vi "PathSettings.vi"() -> ()   [LabVIEW 2010]
uses:
  <vilib>/Utility/config.llb/NI_LVConfig.lvlib
  <vilib>/Utility/config.llb/Read Key (String).vi
panel:
  out "Result: XML Footer":string
  out "Result: XML Header":string
  out "Indicator TAG":string
  out "Control TAG":string
  out "Experiment VI":string
  out "Database":string
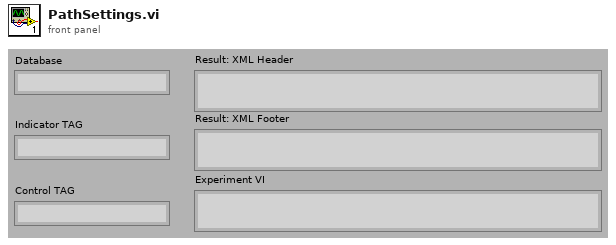
[diagram p1: front panel]
types:
  T1 = typedef "NI_LVConfig.lvlib/Config Data RefNum.ctl" = refnum<k1>
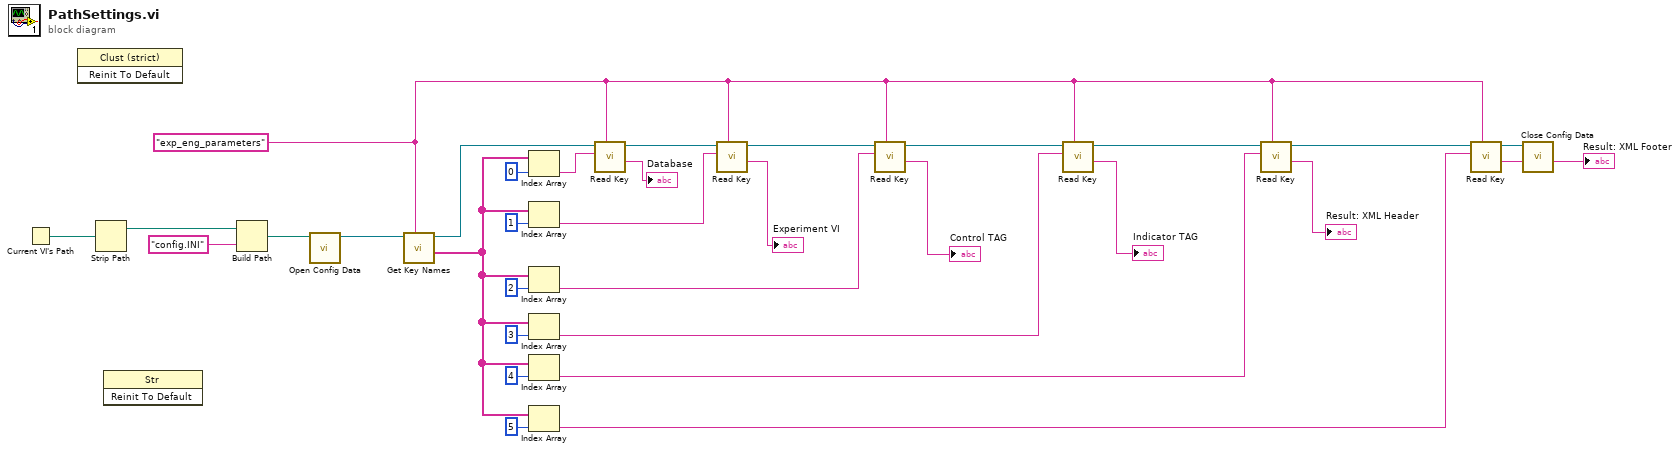
[diagram p0: block diagram]
diagram:
  w9 = "exp_eng_parameters" ("section")
  n1 = Current VI's Path() -> (path=w32:path)
  n2 = invoke on="Invoke Node" class="Clust (strict)" method="Reinit To Default"() -> ()  [unwired: 3 in, 3 out]
  n3 = Strip Path(path=w32) -> (stripped path=w31:path)  [unwired: 1 out]
  n4 = invoke on="Invoke Node" class="Str" method="Reinit To Default"() -> ()  [unwired: 3 in, 3 out]
  n5 = Build Path(base path=w31, name or relative path="config.INI") -> (appended path=w30:path)
  n6 = call <vilib>:"Open Config Data.vi"("configuration file path"=w30) -> ("refnum"=w28:T1)  [unwired: 8 in, 2 out]
  n7 = call <vilib>:"Get Key Names.vi"("section"=w9, "refnum"=w28) -> ("key names"=w11:string[], "refnum out"=w27:T1)  [unwired: 6 in, 2 out]
  n8 = Index Array(array=w11, index=0) -> (element=w25:string)
  n9 = Index Array(array=w11, index=1) -> (element=w23:string)
  n10 = Index Array(array=w11, index=2) -> (element=w19:string)
  n11 = Index Array(array=w11, index=3) -> (element=w16:string)
  n12 = Index Array(array=w11, index=4) -> (element=w14:string)
  n13 = Index Array(array=w11, index=5) -> (element=w10:string)
  n14 = call-poly <vilib>:"Read Key.vi"("section"=w9, "key"=w25, "refnum"=w27) -> ("value"=→"Database":string, "refnum out"=w22:T1)  [unwired: 5 in, 2 out]
  n15 = call-poly <vilib>:"Read Key.vi"("section"=w9, "key"=w23, "refnum"=w22) -> ("value"=→"Experiment VI":string, "refnum out"=w20:T1)  [unwired: 5 in, 2 out]
  n16 = call-poly <vilib>:"Read Key.vi"("section"=w9, "key"=w19, "refnum"=w20) -> ("value"=→"Control TAG":string, "refnum out"=w17:T1)  [unwired: 5 in, 2 out]
  n17 = call-poly <vilib>:"Read Key.vi"("section"=w9, "key"=w16, "refnum"=w17) -> ("value"=→"Indicator TAG":string, "refnum out"=w13:T1)  [unwired: 5 in, 2 out]
  n18 = call-poly <vilib>:"Read Key.vi"("section"=w9, "key"=w14, "refnum"=w13) -> ("value"=→"Result: XML Header":string, "refnum out"=w8:T1)  [unwired: 5 in, 2 out]
  n19 = call-poly <vilib>:"Read Key.vi"("section"=w9, "key"=w10, "refnum"=w8) -> ("value"=→"Result: XML Footer":string, "refnum out"=w7:T1)  [unwired: 5 in, 2 out]
  n20 = call <vilib>:"Close Config Data.vi"("refnum"=w7) -> ()  [unwired: 9 in, 2 out]
